vi "StatePattern_Main.vi"() -> ()   [LabVIEW 2020]
uses:
  State_class/State.lvclass
  NoMoneyState_class/NoMoneyState.lvclass
  C:/Projects/OpenGDS_DesignPatterns/State1/State_class/State.lvclass
  <vilib>/addons/GOOPUtility/GOOPUtility.lvlib
panel:
  out "Class Name":string
  out "GumBalls":i32
  in  "ErrorIn":errorcluster
  out "ErrorOut":errorcluster
  in  "Eject Money":bool
  in  "Turn Crank":bool
  in  "Insert Money":bool
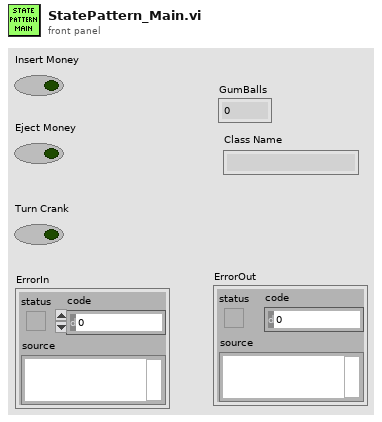
[diagram p1: front panel]
types:
  T1 = cluster{"GumBalls":i32, "Cancelled":bool, "State":refnum<class "State.lvclass">}
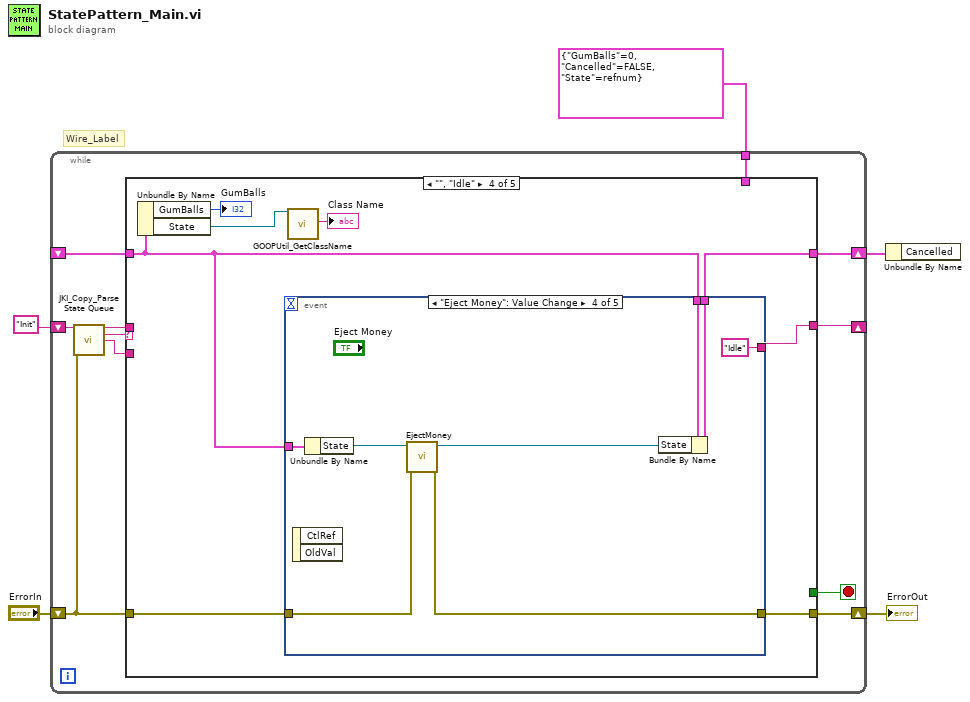
[diagram p0: block diagram]
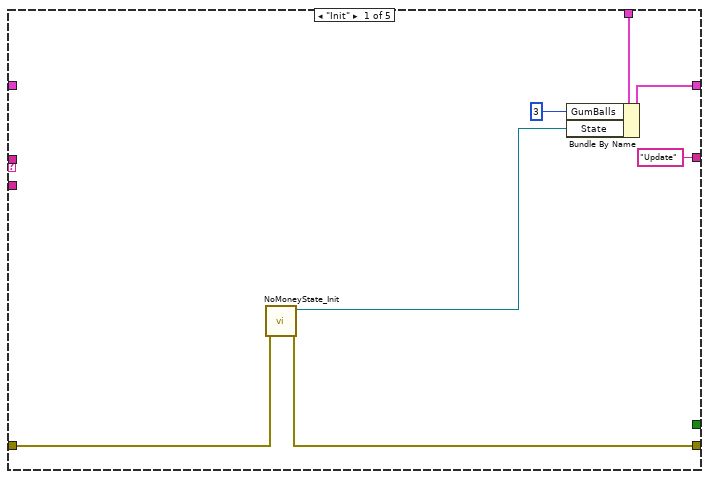
[diagram p2: hidden frame]
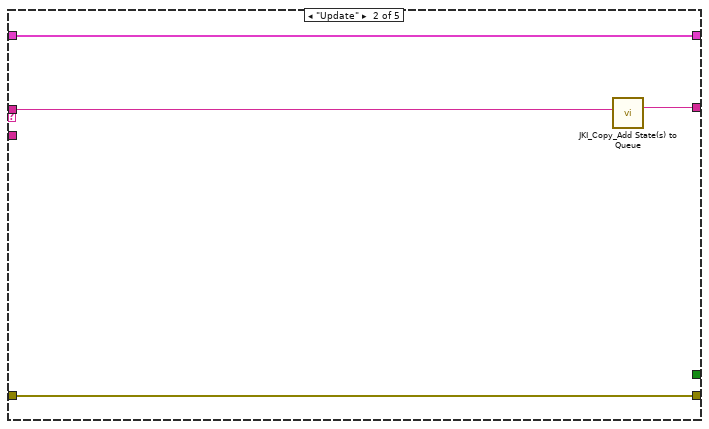
[diagram p3: hidden frame]
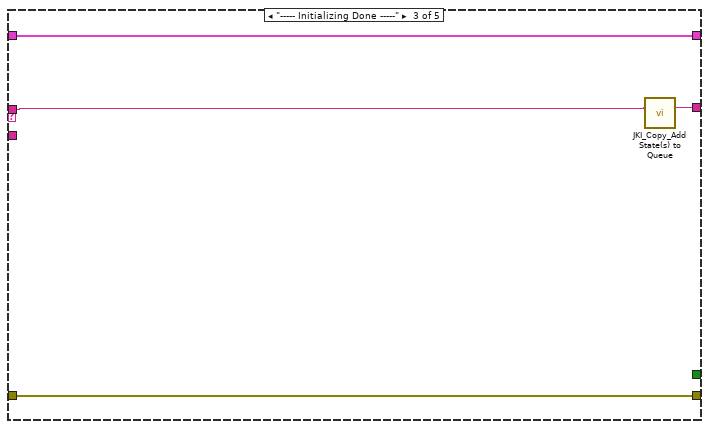
[diagram p4: hidden frame]
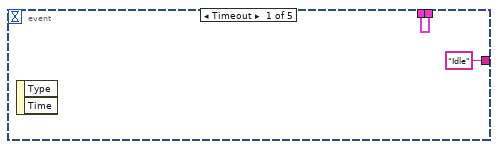
[diagram p5: hidden frame]
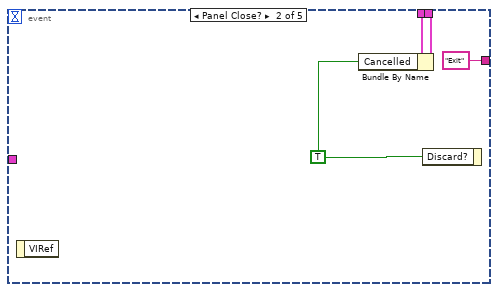
[diagram p6: hidden frame]
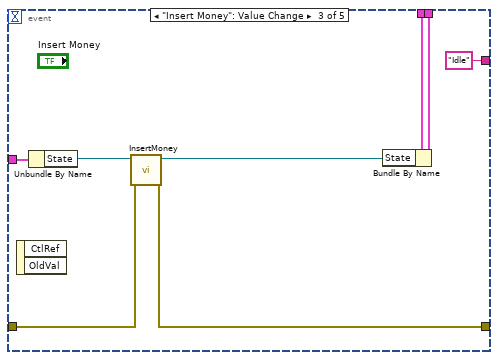
[diagram p7: hidden frame]
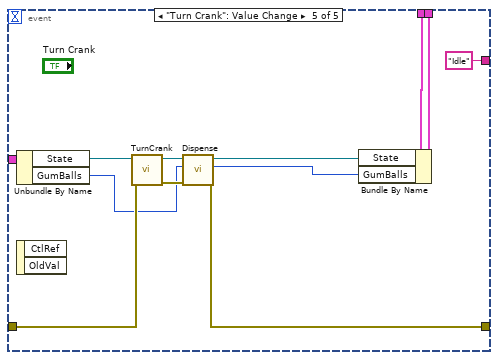
[diagram p8: hidden frame]
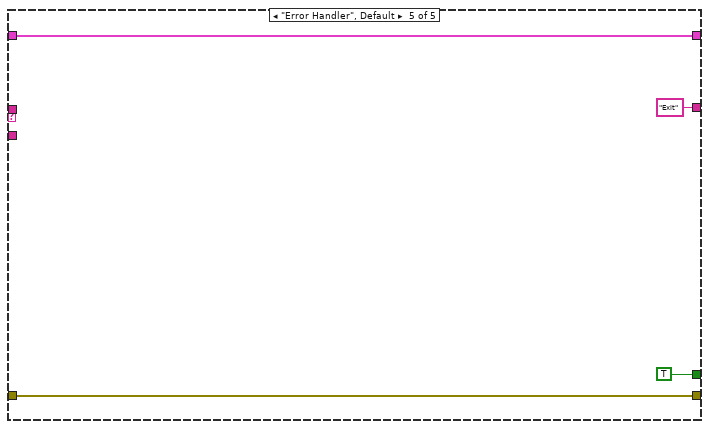
[diagram p9: hidden frame]
diagram:
  # "Wire_Label"
  n1 = while {
    shift-right: [w16] -> w4
    shift-left: "ErrorIn" -> [w7]
    shift-right: [w8] -> _
    shift-left: "Init" -> [w13]
    shift-right: [w15] -> w3
    shift-left: _ -> [w14]
    tunnel: T1 {"GumBalls"=0, "Cancelled"=FALSE, "State"=refnum} -> [w10]
    stop <- w6 stop-if-true
    n2 = call <vilib>:"JKI_Copy_Parse State Queue.vi"("State Queue"=w13, "Error In (no error)"=w7) -> ("Remaining States"=w9:string, "Current State"=w12:string, "Arguments"=w11:string)  [unwired: 11 in]
    n3 = case shown="\"\", \"Idle\"" w12 {
      tunnel: w7 -> [w18 w26 w30 w37 w77]
      tunnel: [w17 w26 w30 w36 w77] -> w16
      tunnel: [w23 w27 w31 w39 w76] -> w15
      tunnel: w14 -> [_ w27 w31 w35 w76]
      tunnel: w11 -> [_ _ _ _ _]
      tunnel: w10 -> [w21 _ _ _ _]
      tunnel: w9 -> [_ w25 w29 _ _]
      tunnel: ["Update" w24 w28 w38 "Exit"] -> w8
      tunnel: [_ _ _ _ TRUE] -> w6
      frame "Init" {
        n4 = call "NoMoneyState_Init.vi"("error in (no error)"=w18) -> ("error out"=w17:errorcluster, "object out"=w19:refnum<class "NoMoneyState.lvclass">)  [unwired: 9 in]
        n5 = Bundle By Name(cluster=w21, "GumBalls"=3 ("Counter"), "State"=w19) -> (w23:T1)
      }
      frame "Update" {
        n6 = call <vilib>:"JKI_Copy_Add State(s) to Queue.vi"("State(s) in (\"\")"=w25) -> ("States Out"=w24:string)  [unwired: 14 in]
      }
      frame "----- Initializing Done -----" {
        n7 = call <vilib>:"JKI_Copy_Add State(s) to Queue.vi"("State(s) in (\"\")"=w29) -> ("States Out"=w28:string)  [unwired: 14 in]
      }
      frame "", "Idle" {
        n8 = Unbundle By Name(w35) -> ("GumBalls"=→"GumBalls":i32, "State"=w33:refnum<class "State.lvclass">)
        n9 = event shown="[3] \"Eject Money\": Value Change" {
          selector: _ -> [_ _ _ _ _]
          dyn-events: _ -> [_ _ _ _ _]
          timeout: _ -> [_ _ _ _ _]
          tunnel: w35 -> [w41 w44 w50 w58 w70]
          tunnel: [w41 w43 w49 w57 w69] -> w39
          tunnel: ["Idle" "Exit" "Idle" "Idle" "Idle"] -> w38
          tunnel: w35 -> [_ _ w53 w61 w73]
          tunnel: w37 -> [_ _ w51 w59 w71]
          tunnel: [_ _ w47 w55 w64] -> w36
          event Timeout {
            n10 = event-data() -> ()  [unwired: 3 out]
          }
          event Panel Close? {
            w42 = TRUE ("Discard?")
            n11 = event-data() -> ()  [unwired: 2 out]
            n12 = Bundle By Name(cluster=w44, "Cancelled"=w42) -> (w43:T1)
            n13 = event-data("Discard?"=w42) -> ()  [unwired: 1 in, 1 out]
          }
          event "Insert Money": Value Change {
            n14 = event-data() -> ()  [unwired: 3 out]
            n15 = Unbundle By Name(w53) -> ("State"=w52:refnum<class "State.lvclass">)
            n16 = call-dynamic "InsertMoney.vi"("error in (no error)"=w51, "object in"=w52) -> ("error out"=w47:errorcluster, "object out"=w46:refnum<class "State.lvclass">)  [unwired: 8 in]
            n17 = Bundle By Name(cluster=w50, "State"=w46) -> (w49:T1)
          }
          event "Eject Money": Value Change {
            n18 = event-data() -> ()  [unwired: 3 out]
            n19 = Unbundle By Name(w61) -> ("State"=w60:refnum<class "State.lvclass">)
            n20 = call-dynamic "EjectMoney.vi"("error in (no error)"=w59, "object in"=w60) -> ("error out"=w55:errorcluster, "object out"=w54:refnum<class "State.lvclass">)  [unwired: 8 in]
            n21 = Bundle By Name(cluster=w58, "State"=w54) -> (w57:T1)
          }
          event "Turn Crank": Value Change {
            n22 = Unbundle By Name(w73) -> ("State"=w72:refnum<class "State.lvclass">, "GumBalls"=w63:i32)
            n23 = event-data() -> ()  [unwired: 3 out]
            n24 = call-dynamic "TurnCrank.vi"("error in (no error)"=w71, "object in"=w72) -> ("error out"=w65:errorcluster, "object out"=w67:refnum<class "State.lvclass">)  [unwired: 8 in]
            n25 = call-dynamic "Dispense.vi"("error in (no error)"=w65, "BallsIn"=w63, "object in"=w67) -> ("error out"=w64:errorcluster, "BallsOut"=w62:i32, "object out"=w66:refnum<class "State.lvclass">)  [unwired: 6 in]
            n26 = Bundle By Name(cluster=w70, "State"=w66, "GumBalls"=w62) -> (w69:T1)
          }
        }
        n27 = call <vilib>:"GOOPUtil_GetClassName.vi"("LabVIEW Object"=w33) -> ("Class Name"=→"Class Name":string)  [unwired: 14 in, 4 out]
      }
      frame "Error Handler", Default {
      }
    }
  }
  "ErrorOut" <- w4
  n28 = Unbundle By Name(w3) -> ()  [unwired: 1 out]
